vi "UpdateSelectROIOverlay.vi"(8 "error in (no error)":errorcluster, 10 "Index":i32, 11 "Image Refnum":refnum<vi>) -> (0 "error out":errorcluster)   [LabVIEW 2019]
uses:
  Controls/ROI_List_Action.ctl
  <vilib>/vision/Image Controls.llb/IMAQ Image.ctl
panel:
  in  "Vision_Image":T1(plugin-control)
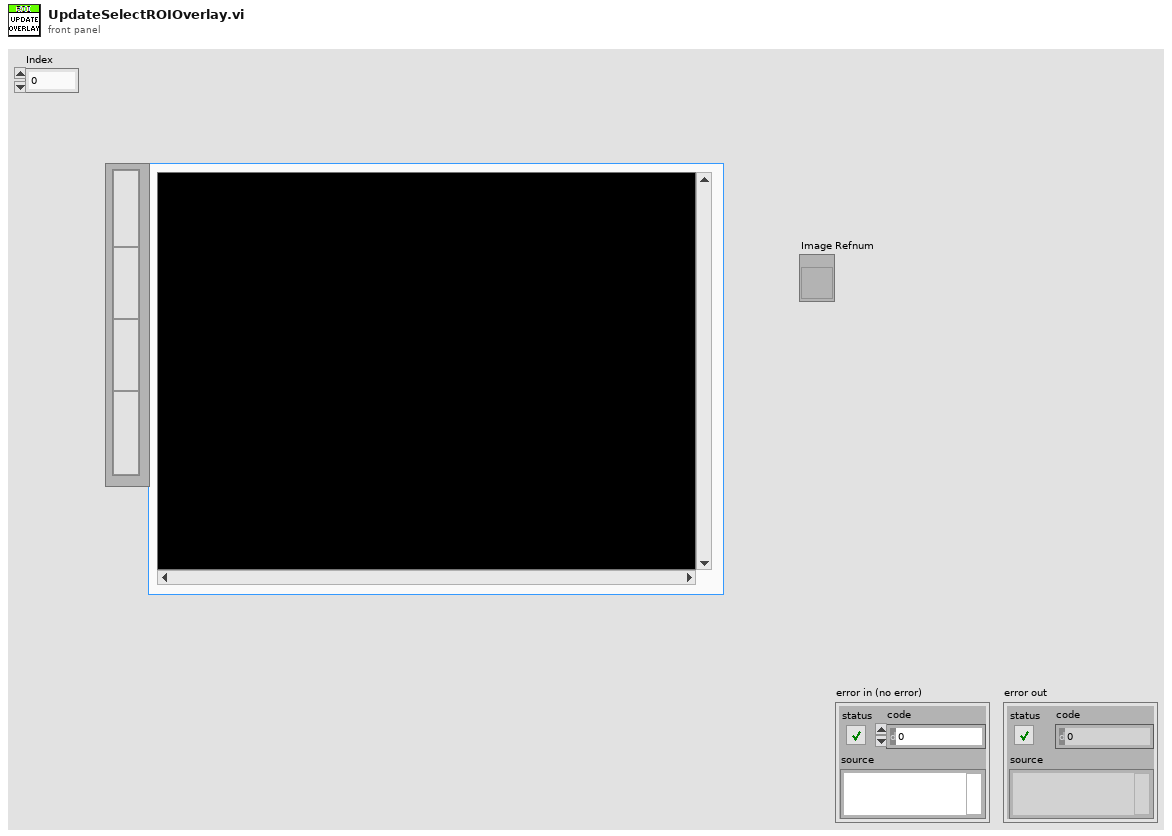
[diagram p1: front panel]
types:
  T1 = typedef "IMAQ Image.ctl" = refnum<image>
  T2 = typedef "ROI_List_Action.ctl" = enum16{"Init", "Add ROI", "Delete ROI", "Get All ROI", "Get Specific ROI", "Set Analysis Setting", "Set Process Setting", "Replace All Entries", "ROIEntryBackup", "ROIEntryBackupClear", "ROIEntryReturn"}
  T3 = typedef "Vision_DataEntry.ctl" = cluster{"vROIName":string, "vROIContour":cluster{"Contour Type":u32, "ROI Type":u32, "Points":i32[]}, "ProcessSetting":T4[], "Analysis_Setting":T6}
  T4 = typedef "Process_Setting.ctl" = cluster{"Enum_PreProcess":T5, "Parameter":string}
  T5 = typedef "VisionProcessName.ctl" = enum16{"*CamParameter*", "CamAttributes", "*Preprocess*", "CG_Brightness", "C_Plane Extraction", "C_Threshold", "G_Lookup Table", "G_Threshold"}
  T6 = typedef "Analysis_Setting.ctl" = cluster{"PreProcess":T7, "Parameter":string}
  T7 = typedef "V_Analysis_Type.ctl" = enum16{"None", "C_Color Pattern Matching", "G_PatternMatching", "G_ShapeDectect", "G_GeometricMatch", "B_Area Check"}
  T8 = cluster{"Points[0]":i32, "Points[1]":i32, "Points[2]":i32, "Points[3]":i32}
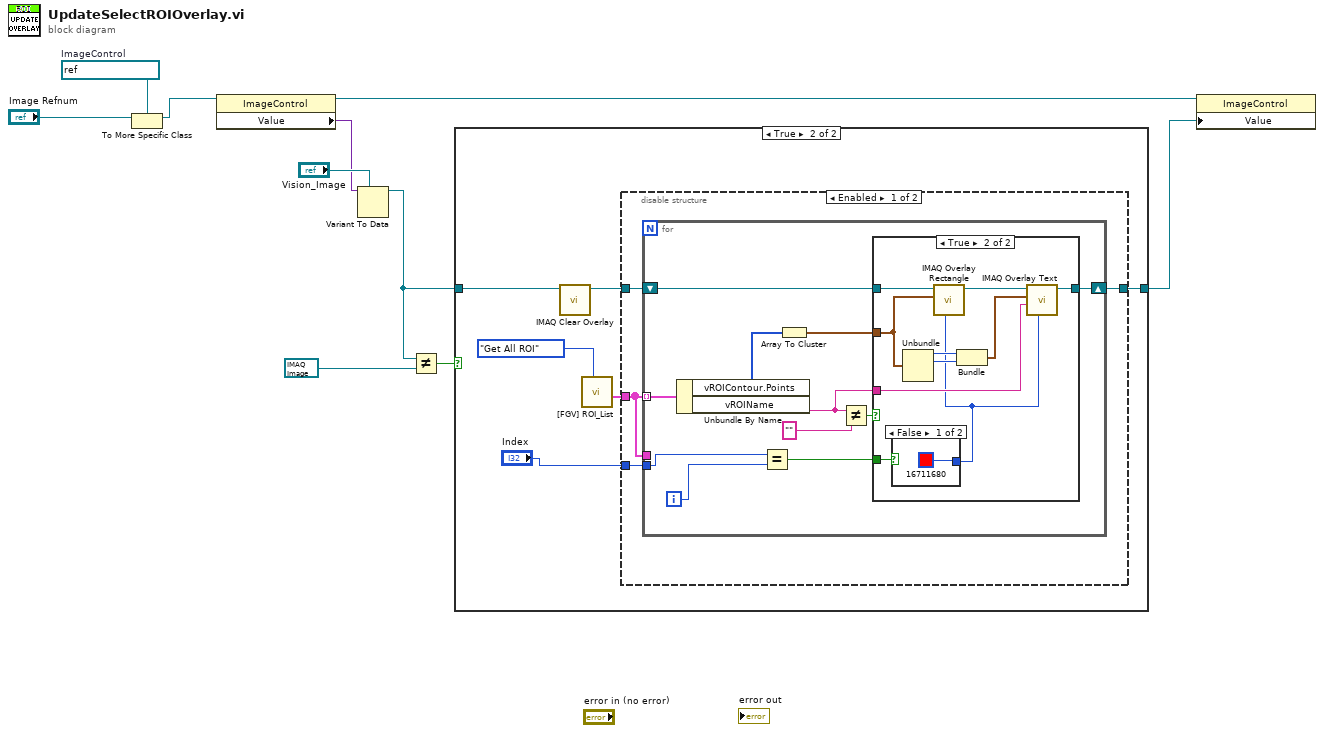
[diagram p0: block diagram]
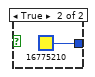
[diagram p4: hidden frame]
diagram:
  w9 = refnum<vi> refnum  # ImageControl
  n1 = To More Specific Class(target class=w9, reference="Image Refnum") -> (specific class reference=w8:refnum<vi>)  [unwired: 1 in, 1 out]
  n2 = property class="ImageControl"(reference=w8) -> (reference out=w7:refnum<vi>, "Value"=w4:variant)  [unwired: 1 in, 1 out]
  n3 = Variant To Data(type="Vision_Image", Variant=w4) -> (data=w3:T1)  [unwired: 1 in, 1 out]
  n4 = Not Equal?(x=w3, y=T1 refnum ("Image Out")) -> (x != y?=w1:bool)
  n5 = case shown="True" w1 {
    tunnel: [w11 w15] -> w6
    tunnel: w3 -> [w11 w14]
    frame False {
    }
    frame True {
      n6 = call "IMAQ Clear Overlay"("Image"=w14) -> ("Image Out"=w13:T1)  [unwired: 9 in, 1 out]
      n7 = call "[FGV] ROI_List.vi"("Action"=ROI_List_Action."Get All ROI") -> ("All ROI"=w16:T3[])  [unwired: 8 in, 2 out]
      n8 = disable-structure shown="Enabled" {
        disable-tunnel: w16 -> [w19 _]
        disable-tunnel: w13 -> [w21 _]
        disable-tunnel: [w20 _] -> w15
        disable-tunnel: "Index" -> [w18 _]
        frame Enabled {
          n9 = for {
            tunnel: w19 -> [w30] mode=indexing
            shift-right: [w31] -> w20
            shift-left: w21 -> [w32]
            tunnel: w19 -> [_]
            tunnel: w18 -> [w22]
            i -> [w23]
            n10 = Unbundle By Name(w30) -> ("vROIContour.Points"=w27:i32[], "vROIName"=w25:string)
            n11 = Equal?(x=w22, y=w23) -> (x = y?=w24:bool)
            n12 = Array To Cluster(array=w27) -> (cluster=w26:T8)
            n13 = Not Equal?(x=w25, y="") -> (x != y?=w28:bool)
            n14 = case shown="True" w28 {
              tunnel: w32 -> [w33 w43]
              tunnel: [w33 w41] -> w31
              tunnel: w26 -> [_ w39]
              tunnel: w25 -> [_ w40]
              tunnel: w24 -> [_ w35]
              frame False {
              }
              frame True {
                n15 = case shown="False" w35 {
                  tunnel: [u32 16711680 ("Text Color (black)") u32 16775210 ("Text Color (black)")] -> w34
                  frame False {
                  }
                  frame True {
                  }
                }
                n16 = Unbundle(w39) -> ("Points[0]"=w38:i32, "Points[1]"=w37:i32)  [unwired: 2 out]
                n17 = call "IMAQ Overlay Rectangle"("Color"=w34, "Rectangle"=w39, "Image"=w43) -> ("Image Out"=w42:T1)  [unwired: 7 in, 1 out]
                n18 = Bundle("Points[0]"=w38, "Points[1]"=w37) -> (w36:cluster{"Points[0]":i32, "Points[1]":i32})  [unwired: 1 in]
                n19 = call "IMAQ Overlay Text"("Text Color (black)"=w34, "String"=w40, "Origin"=w36, "Image"=w42) -> ("Image Out"=w41:T1)  [unwired: 6 in, 1 out]
              }
            }
          }
        }
        frame Disabled {
        }
      }
    }
  }
  n20 = property class="ImageControl"(reference=w7, "Value"=w6) -> ()  [unwired: 1 in, 2 out]
